vi "zern2slopes.vi"(7 "idxType":enum16{"Wyant", "ANSI"}(ring), 8 "error in (no error)":errorcluster, 9 "Zern coef in":sgl[](array[numeric]), 10 "Zern index in":i32[](array[numeric]), 11 "HasoSlopes in":refnum<class "HasoSlopes.lvclass">) -> (0 "error out":errorcluster, 1 "Zern pupil out":refnum<class "Pupil.lvclass">, 2 "ModalCoef out":refnum<class "ModalCoef.lvclass">, 3 "HasoSlopes out":refnum<class "HasoSlopes.lvclass">)   [LabVIEW 2018]
uses:
  <userlib>/WaveKit.lib/Controls/HasoSlopes.lvclass
  <userlib>/WaveKit.lib/Classes/ModalCoef/ModalCoef.lvclass
  <userlib>/WaveKit.lib/Controls/Pupil.lvclass
  <userlib>/WaveKit.lib/Controls/WavefrontModalReconstructionType.ctl
  <userlib>/WaveKit.lib/Controls/ZernikeModalPrefs.ctl
  <userlib>/WaveKit.lib/Controls/ZernikeProjectionPupilSetup.ctl
  <userlib>/WaveKit.lib/Controls/Point2Df.ctl
  <userlib>/WaveKit.lib/Controls/CircularPupilDetectionParams.ctl
  <userlib>/WaveKit.lib/Controls/PupilDetectionOption.ctl
  <userlib>/WaveKit.lib/Controls/CircularAutoDetectionOptions.ctl
  <userlib>/WaveKit.lib/Controls/PupilDetectionMode.ctl
  <userlib>/WaveKit.lib/Classes/ComputePhaseSet/ComputePhaseSet.lvclass
  <userlib>/WaveKit.lib/Controls/WavefrontReconstructionMode.ctl
panel:
  # "Zern index in: 1D array, no more than 32 elements, each element value 1~32\nZern coef in: 1D array, coefficients corresponding to the indexes in Zern index in"
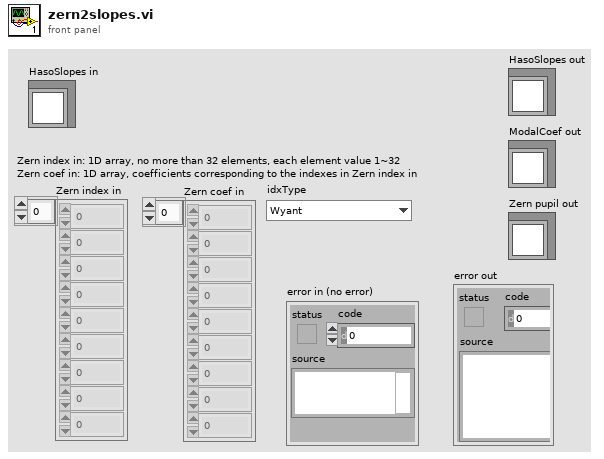
[diagram p1: front panel]
types:
  T1 = typedef "WavefrontReconstructionMode.ctl" = enum16{"None", "Modal_Legendre", "Modal_Zernike", "Zonal", "Modal_Zonal_Zernike", "Modal_Zonal_Legendre"}
  T2 = typedef "CircularPupilDetectionParams.ctl" = cluster{"PupilDetectionOption":T3, "AutoDetectionOption":T4, "PupilDetectionMode":T5, "CentralOccultationDetection":bool}
  T3 = typedef "PupilDetectionOption.ctl" = enum16{"Manual", "Automatic"}
  T4 = typedef "CircularAutoDetectionOptions.ctl" = enum16{"manual_radius_auto_center", "manual_center_auto_radius", "auto_radius_auto_center"}
  T5 = typedef "PupilDetectionMode.ctl" = enum16{"inscribed", "circumscribed"}
  T6 = typedef "ZernikeModalPrefs.ctl" = cluster{"Number of coefficients":u32, "Filtered coefficients":u32[], "RMS Zernike normalization":bool, "CircularProjectionPupilDimensions":T7}
  T7 = typedef "ZernikeProjectionPupilSetup.ctl" = cluster{"Pupil center_sspp":T8, "Pupil radius_sspp":sgl}
  T8 = typedef "Point2Df.ctl" = cluster{"X":sgl, "Y":sgl}
  T9 = typedef "WavefrontModalReconstructionType.ctl" = enum16{"Legendre", "Zernike"}
  T10 = enum16{"ANSI2Wyant", "Wyant2ANSI", "ANSI2ANSI", "Wyant2Wyant"}
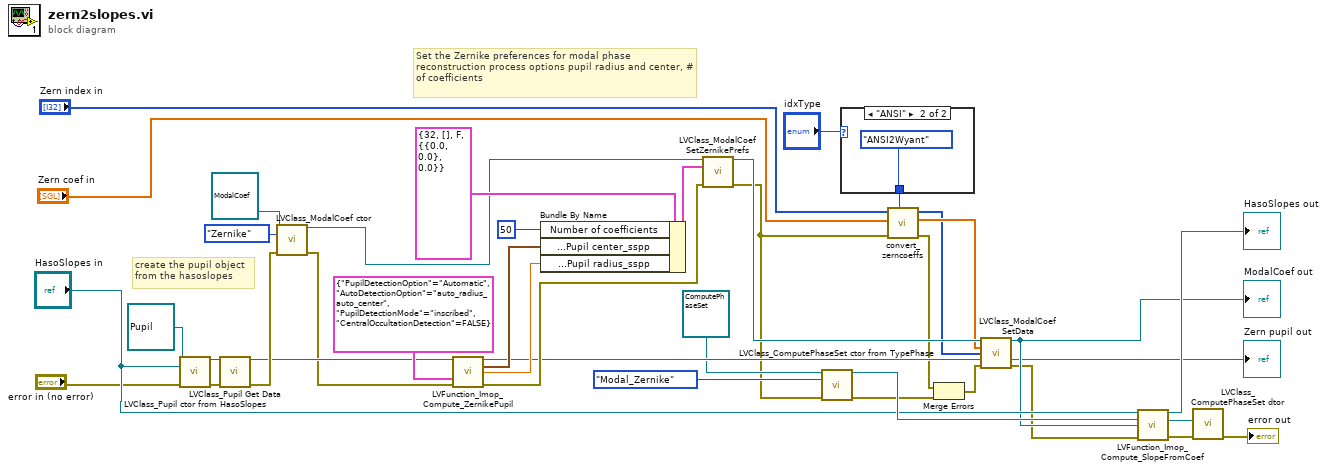
[diagram p0: block diagram]
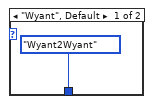
[diagram p2: hidden frame]
diagram:
  # "create the pupil object\nfrom the hasoslopes"
  # "Set the Zernike preferences for modal phase reconstruction process options pupil radius and center, # of coefficients"
  n1 = call <userlib>:"LVClass_Pupil ctor from HasoSlopes.vi"("Pupil in"=refnum<class "Pupil.lvclass"> refnum, "HasoSlopes.lvclass"="HasoSlopes in", "error in (no error)"="error in (no error)") -> ("Pupil out"=w30:refnum<class "Pupil.lvclass">, "error out"=w29:errorcluster)  [unwired: 11 in]
  n2 = call <userlib>:"LVClass_Pupil Get Data.vi"("Pupil in"=w30, "error in (no error)"=w29) -> ("Pupil out"=w27:refnum<class "Pupil.lvclass">, "error out"=w28:errorcluster)  [unwired: 11 in, 1 out]
  n3 = call <userlib>:"LVClass_ModalCoef ctor.vi"("ModalCoef in"=refnum<class "ModalCoef.lvclass"> refnum, "TypePhase"=WavefrontModalReconstructionType."Zernike", "error in (no error)"=w28) -> ("ModalCoef out"=w36:refnum<class "ModalCoef.lvclass">, "error out"=w26:errorcluster)  [unwired: 11 in]
  n4 = call <userlib>:"LVFunction_Imop_Compute_ZernikePupil.vi"("Pupil.lvclass"=w27, "CircularPupilDetectionParams"=T2 {"PupilDetectionOption"=enum."Automatic", "AutoDetectionOption"=enum."auto_radius_auto_center", "PupilDetectionMode"=enum."inscribed", "CentralOccultationDetection"=FALSE}, "error in"=w26) -> ("Pupil.lvclass"=w24:refnum<class "Pupil.lvclass">, "center"=w32:T8, "radius"=w33:sgl, "error out"=w25:errorcluster)  [unwired: 9 in]
  n5 = Bundle By Name(cluster=T6 {"Number of coefficients"=32, "Filtered coefficients"=[], "RMS Zernike normalization"=FALSE, "CircularProjectionPupilDimensions"={"Pupil center_sspp"={"X"=0.0, "Y"=0.0}, "Pupil radius_sspp"=0.0}} ("ZernikeModalPrefs"), "Number of coefficients"=u32 50, "CircularProjectionPupilDimensions.Pupil center_sspp"=w32, "CircularProjectionPupilDimensions.Pupil radius_sspp"=w33) -> (w38:T6)
  n6 = call <userlib>:"LVClass_ModalCoef SetZernikePrefs.vi"("ModalCoef in"=w36, "ZernikeModalPrefs"=w38, "error in (no error)"=w25) -> ("ModalCoef out"=w23:refnum<class "ModalCoef.lvclass">, "error out"=w6:errorcluster)  [unwired: 11 in]
  n7 = call <userlib>:"LVClass_ComputePhaseSet ctor from TypePhase.vi"("ComputePhaseSet in"=refnum<class "ComputePhaseSet.lvclass"> refnum, "TypePhase"=WavefrontReconstructionMode."Modal_Zernike", "error in (no error)"=w6) -> ("ComputePhaseSet out"=w20:refnum<class "ComputePhaseSet.lvclass">, "error out"=w9:errorcluster)  [unwired: 11 in]
  n8 = case shown="\"ANSI\"" "idxType" {
    tunnel: [T10."Wyant2Wyant" ("ConType") T10."ANSI2Wyant" ("ConType")] -> w1
    frame "Wyant", Default {
    }
    frame "ANSI" {
    }
  }
  n9 = call "convert_zerncoeffs.vi"("ConType"=w1, "error in (no error)"=w6, "Zern coef in"="Zern coef in", "Zern indx in"="Zern index in") -> ("error out"=w5:errorcluster, "Zern Coef Out"=w4:dbl[], "Zern index out"=w3:i32[])  [unwired: 5 in]
  n10 = Merge Errors(w5, w9) -> (w10:errorcluster)
  n11 = call <userlib>:"LVClass_ModalCoef SetData.vi"("ModalCoef in"=w23, "coef"=w4, "index"=w3, "Pupil.lvclass"=w24, "error in (no error)"=w10) -> ("ModalCoef out"=w14:refnum<class "ModalCoef.lvclass">, "Pupil (dup)"=→"Zern pupil out":refnum<class "Pupil.lvclass">, "error out"=w13:errorcluster)  [unwired: 7 in, 1 out]
  "ModalCoef out" <- w14
  n12 = call <userlib>:"LVFunction_Imop_Compute_SlopeFromCoef.vi"("HasoSlopes.lvclass"="HasoSlopes in", "ComputePhaseSet"=w20, "ModalCoef.lvclass"=w14, "error IO"=w13) -> ("HasoSlopes.lvclass"=→"HasoSlopes out":refnum<class "HasoSlopes.lvclass">, "ComputePhaseSet (dup)"=w19:refnum<class "ComputePhaseSet.lvclass">, "error IO out"=w16:errorcluster)  [unwired: 8 in, 1 out]
  n13 = call <userlib>:"LVClass_ComputePhaseSet dtor.vi"("ComputePhaseSet in"=w19, "error in (no error)"=w16) -> ("error out"=→"error out":errorcluster)  [unwired: 12 in, 1 out]
